vi "Main.vi"() -> ()   [LabVIEW 2014, in "5. Creating a User-Defined Signal.lvlib"]
doc: "In the previous example, \"4. Inheriting from a Widget\", we encapsulated the slider inside the Number Widget. As a result, the outside world no longer has access to the signals emitted by the slider.\n\nTo compensate, this example adds a user-defined signal to the Number Widget. We make connections in such a way that our newly-defined signal lets us respond to changes in the encapsulated slider.\n\n\n<b>Showcase</b>\n- Creating user-defined signals\n- Connecting one signal to another signal (a.k.a. Relaying)\n\n\nCopyright (c) 2019 Sze Howe Koh.\nThis code is licensed under the MIT license."
uses:
  5. Creating a User-Defined Signal.lvlib
  <vilib>/addons/LQ/LQ Core/QSize.ctl
  <vilib>/addons/LQ/Qt Widgets/QWidget/resize.vi
  <vilib>/addons/LQ/Qt Widgets/QWidget/setVisible.vi
  <vilib>/addons/LQ/LQ Core/LQCoreEngine/_Polymorphic Instances/Connect_EventRefOut_DBL.vi
  <vilib>/addons/LQ/LQ Core/LQCoreEngine/LQCoreEngine.lvclass
  Number Widget/Number Widget.lvclass
panel:
  out "Widget Value":dbl
  in  "Stop Button":bool
  # "Prerequisite knowledge/experience\n- Example 3b. Connecting a Signal to a LabVIEW Event\n- Example 4. Inheriting from a Widget\n\n\nDescription\nIn the previous example, 4. Inheriting from a Widget, we encapsulated the slider inside the Number\nWidget. As a result, the outside world no longer has access to the signals emitted by the slider.\n\nTo compensate, this example adds a user-defined signal to the Number Widget. We make connections\nin such a way that our newly-defined signal lets us respond to changes in the encapsulated slider.\n\n\nShowcase\n- Creating user-defined signals\n- Connecting one signal to another signal (a.k.a. Relaying)"
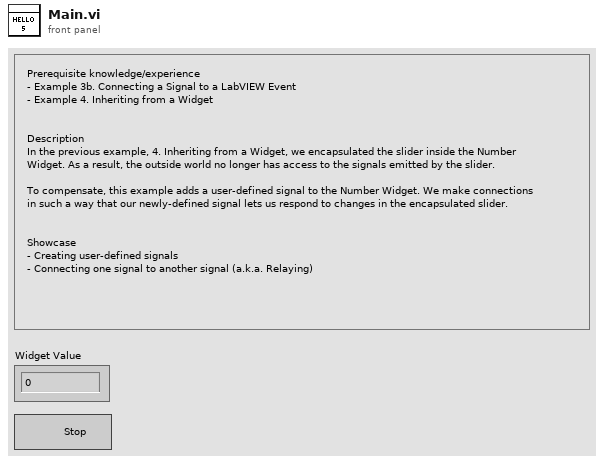
[diagram p1: front panel]
types:
  T1 = typedef "QSize.ctl" = cluster{"width":i32, "height":i32}
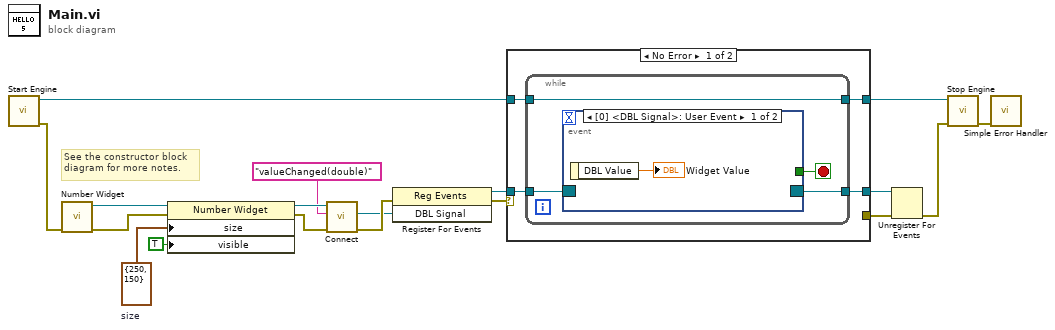
[diagram p0: block diagram]
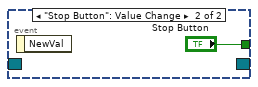
[diagram p2: hidden frame]
diagram:
  w17 = T1 {"width"=250, "height"=150}  # size
  # "See the constructor block\ndiagram for more notes."
  n1 = call <vilib>:"Start Engine.vi"() -> ("Error Out"=w14:errorcluster, "New Engine"=w5:refnum<class "LQCoreEngine.lvclass">)  [unwired: 10 in]
  n2 = call "Number Widget.vi"("Error In"=w14) -> ("Error Out"=w13:errorcluster, "New Number Widget"=w15:refnum<class "Number Widget.lvclass">)  [unwired: 9 in]
  n3 = property class="Number Widget"(reference=w15, error in=w13, "size"=w17, "visible"=TRUE) -> (reference out=w4:refnum<class "Number Widget.lvclass">, error out=w8:errorcluster)
  n4 = call-poly <vilib>:"Connect.vi"("Error In"=w8, "Signal Signature"="valueChanged(double)", "Sender In"=w4) -> ("Error Out"=w9:errorcluster, "DBL Signal"=w3:refnum<user-event>)  [unwired: 6 in, 1 out]
  n5 = register-events(error in=w9, w3) -> (reference out=w12:refnum<event-registration>, error out=w2:errorcluster)  [unwired: 1 in]
  n6 = case shown="No Error" w2 {
    selector: w2 -> [_ w29]
    tunnel: w5 -> [w22 w31]
    tunnel: [w21 w31] -> w6
    tunnel: w12 -> [w20 w30]
    tunnel: [w19 w30] -> w11
    tunnel: [_ w29] -> w10
    frame No Error {
      n7 = while {
        tunnel: w20 -> [w25]
        tunnel: [w23] -> w19
        tunnel: w22 -> [w26]
        tunnel: [w26] -> w21
        stop <- w24 stop-if-true
        n8 = event shown="[0] <DBL Signal>: User Event" {
          selector: w25 -> [_ _]
          dyn-events: [_ _] -> w23
          timeout: _ -> [_ _]
          tunnel: [_ "Stop Button"] -> w24
          event User Event {
            n9 = event-data() -> ("DBL Value"=→"Widget Value":dbl)  [unwired: 1 in]
          }
          event "Stop Button": Value Change {
            n10 = event-data() -> ()  [unwired: 1 in, 1 out]
          }
        }
      }
    }
    frame Error {
    }
  }
  n11 = Unregister For Events(event registration refnum=w11, error in=w10) -> (error out=w7:errorcluster)
  n12 = call <vilib>:"Stop Engine.vi"("Error In"=w7, "LQCoreEngine"=w6) -> ("Error Out"=w18:errorcluster)  [unwired: 9 in]
  n13 = call <vilib>:"Simple Error Handler.vi"("error in (no error)"=w18) -> ()  [unwired: 4 in, 5 out]
